vi "Write Elevator Position.vi"(8 "error in (no error)":errorcluster, 10 "Elevator Position":T1, 11 "Sim Sensor Interface in":refnum<class "Sim Sensor Interface.lvclass">) -> (0 "error out":errorcluster, 3 "Sim Sensor Interface out":refnum<class "Sim Sensor Interface.lvclass">)   [LabVIEW 2019, in "Simulated Sensor Interface Actor.lvlib" / "Sim Sensor Interface.lvclass"]
uses:
  Sim Sensor Interface.lvclass
  Sim Display Console Actor/Elevator Controller/Floor -Enum.ctl
  Sim Display Console Actor/Elevator Controller/Sim Display Console Actor.lvclass
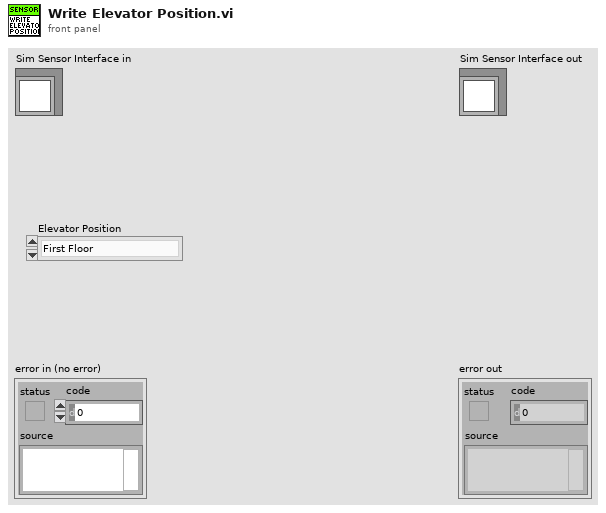
[diagram p1: front panel]
types:
  T1 = typedef "Simulated Display Console Actor.lvlib/Sim Display Console Actor.lvclass/Floor -Enum.ctl" = enum16{"First Floor", "Send Floor", "Third Floor", "Fourth Floor"}
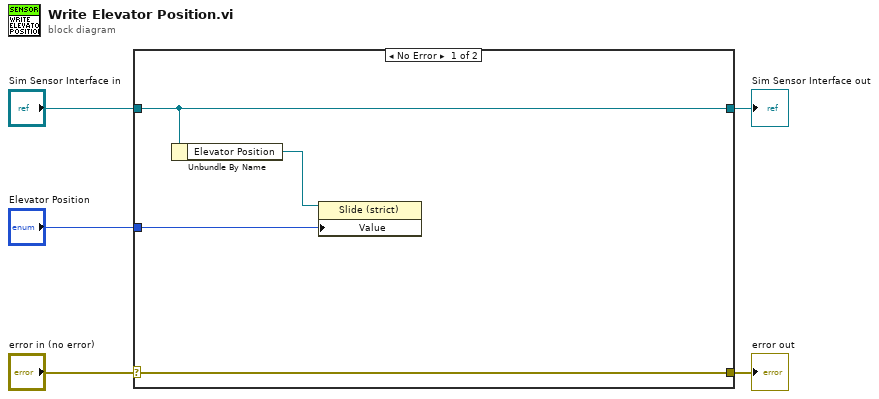
[diagram p0: block diagram]
diagram:
  n1 = case shown="No Error" "error in (no error)" {
    selector: "error in (no error)" -> [w9 w11]
    tunnel: [w9 w11] -> w4
    tunnel: [w8 w10] -> w2
    tunnel: "Sim Sensor Interface in" -> [w8 w10]
    tunnel: "Elevator Position" -> [w6 _]
    frame No Error {
      n2 = Unbundle By Name(w8) -> ("Elevator Position"=w7:refnum<vi>)
      n3 = property class="Slide (strict)"(reference=w7, "Value"=w6) -> ()  [unwired: 1 in, 2 out]
    }
    frame Error {
    }
  }
  "error out" <- w4
  "Sim Sensor Interface out" <- w2
